vi "globalTearDown.vi"(8 "error in (no error)":errorcluster, 11 "testcase-CSMNonCSMCallerSupportAPI in":refnum<class "testcase-CSMNonCSMCallerSupportAPI.lvclass">) -> (0 "error out":errorcluster, 3 "testcase-CSMNonCSMCallerSupportAPI out":refnum<class "testcase-CSMNonCSMCallerSupportAPI.lvclass">)   [LabVIEW 2017, in "testcase-CSMNonCSMCallerSupportAPI.lvclass"]
uses:
  testcase-CSMNonCSMCallerSupportAPI.lvclass
  testcase-CSMNonCSMCallerSupportAPI.lvclass/testcase-CSMNonCSMCallerSupportAPI.ctl
  <vilib>/addons/_JKI Toolkits/VI Tester/TestCase.llb/TestCase.lvclass
  src/user.lib/_NEVSTOP/Communicable State Machine(CSM)/_Support/Typedef/_CSM_List Module Scope.ctl
  src/user.lib/_NEVSTOP/Communicable State Machine(CSM)/Communicable State Machine.lvlib
panel:
  out "CSMs":string[](array[string])
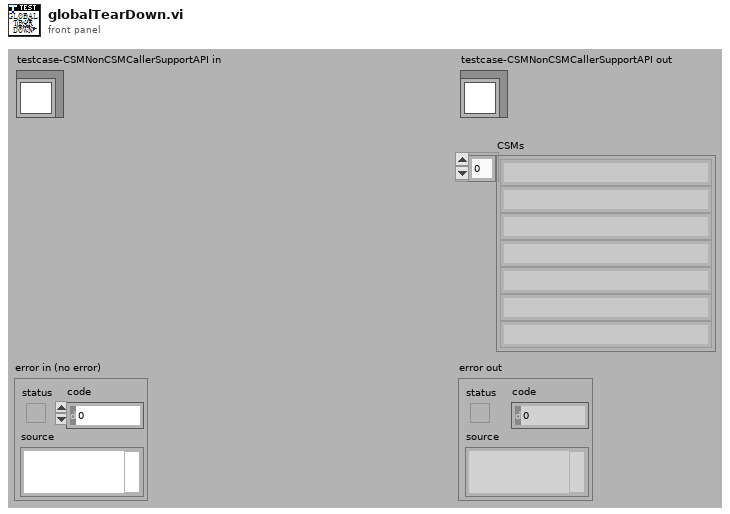
[diagram p1: front panel]
types:
  T1 = typedef "Communicable State Machine.lvlib/_CSM_List Module Scope.ctl" = enum16{"Normal", "System Only", "All"}
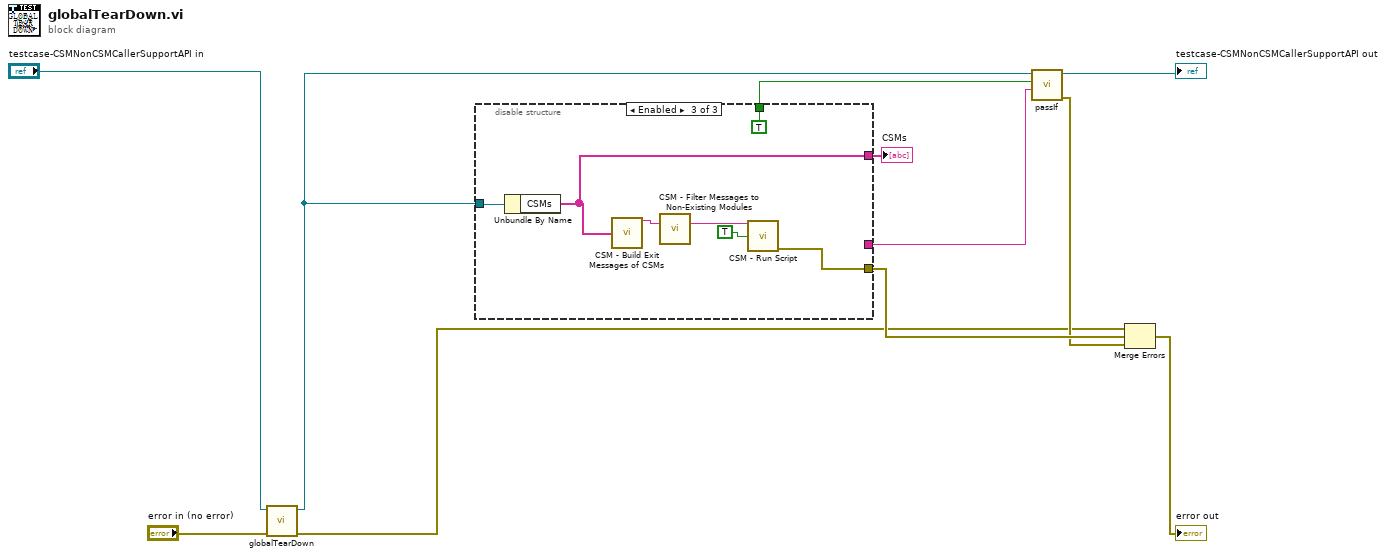
[diagram p0: block diagram]
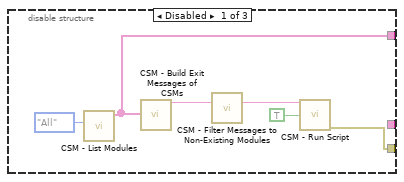
[diagram p2: hidden frame]
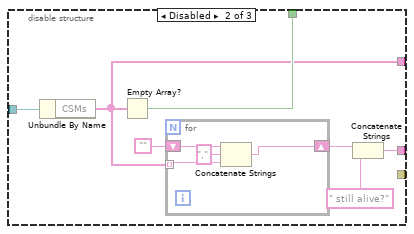
[diagram p3: hidden frame]
diagram:
  n1 = call-parent "globalTearDown.vi"("error in (no error)"="error in (no error)", "TestCase in"="testcase-CSMNonCSMCallerSupportAPI in") -> ("error out"=w5:errorcluster, "TestCase out"=w2:refnum<class "testcase-CSMNonCSMCallerSupportAPI.lvclass">)  [unwired: 8 in]
  n2 = disable-structure shown="Enabled" {
    disable-tunnel: [w13 _ w30] -> w7
    disable-tunnel: w2 -> [_ w24 w35]
    disable-tunnel: [w12 w22 w31] -> w1
    disable-tunnel: [_ w23 TRUE ("pass")] -> w9
    disable-tunnel: [_ w18 _] -> w8
    frame Disabled {
      n3 = call "CSM - List Modules.vi"("Scope (Normal)"=_CSM_List_Module_Scope."All") -> ("Module Names"=w12:string[])  [unwired: 9 in, 1 out]
      n4 = call "CSM - Build Exit Messages of CSMs.vi"("CSMs"=w12) -> ("States"=w17:string)  [unwired: 14 in]
      n5 = call "CSM - Filter Messages to Non-Existing Modules.vi"("States In"=w17) -> ("States Out"=w15:string)  [unwired: 14 in]
      n6 = call "CSM - Run Script.vi"("CSM Scripts"=w15, "Continue If Error? (F)"=TRUE) -> ("error out"=w13:errorcluster)  [unwired: 11 in, 2 out]
    }
    frame Disabled {
      n7 = Unbundle By Name(w24) -> ("CSMs"=w22:string[])
      n8 = Empty Array?(array=w22) -> (empty?=w23:bool)
      n9 = for {
        tunnel: w22 -> [w26] mode=indexing
        shift-right: [w27] -> w20
        shift-left: "" -> [w28]
        n10 = Concatenate Strings(w28, "," ("string"), w26) -> (w27:string)
      }
      n11 = Concatenate Strings(w20, " still alive?" ("string")) -> (w18:string)
    }
    frame Enabled {
      n12 = Unbundle By Name(w35) -> ("CSMs"=w31:string[])
      n13 = call "CSM - Build Exit Messages of CSMs.vi"("CSMs"=w31) -> ("States"=w34:string)  [unwired: 14 in]
      n14 = call "CSM - Filter Messages to Non-Existing Modules.vi"("States In"=w34) -> ("States Out"=w32:string)  [unwired: 14 in]
      n15 = call "CSM - Run Script.vi"("CSM Scripts"=w32, "Continue If Error? (F)"=TRUE) -> ("error out"=w30:errorcluster)  [unwired: 11 in, 2 out]
    }
  }
  "CSMs" <- w1
  n16 = call-dynamic "passIf.vi"("message (\"\")"=w8, "pass"=w9, "TestCase in"=w2) -> ("error out"=w6:errorcluster, "TestCase out"=→"testcase-CSMNonCSMCallerSupportAPI out":refnum<class "testcase-CSMNonCSMCallerSupportAPI.lvclass">)  [unwired: 7 in]
  n17 = Merge Errors(w5, w7, w6) -> (→"error out":errorcluster)
